vi "Abort.vi"(8 "error in (no error)":errorcluster, 11 "WAMP Client in":refnum<class "WAMP Client.lvclass">) -> (0 "error out":errorcluster, 3 "WAMP Client out":refnum<class "WAMP Client.lvclass">)   [LabVIEW 2020, in "wamplv.lvlib" / "WAMP Client.lvclass"]
uses:
  WAMP Client.lvclass
  Private/TypeDefs/WAMP Message Codes.ctl
  WAMP Client.lvclass/WAMP Client.ctl
  Private/Comm Handlers/ICommHandler/ICommHandler.lvclass
  wamplv.lvlib
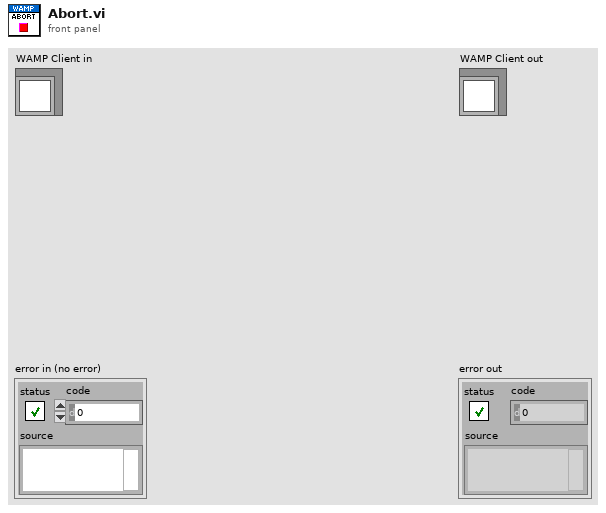
[diagram p1: front panel]
types:
  T1 = typedef "wamplv.lvlib/WAMP Message Codes.ctl" = u16
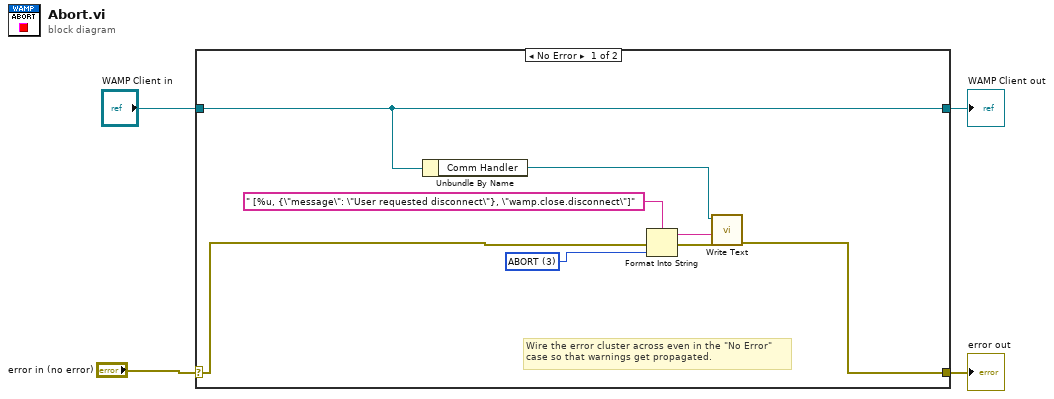
[diagram p0: block diagram]
diagram:
  n1 = case shown="No Error" "error in (no error)" {
    selector: "error in (no error)" -> [w7 w14]
    tunnel: [w5 w14] -> w3
    tunnel: [w12 w13] -> w1
    tunnel: "WAMP Client in" -> [w12 w13]
    frame No Error {
      w10 = T1 3 items=["HELLO"=1, "WELCOME"=2, "ABORT"=3, "GOODBYE"=6, "ERROR"=8, "PUBLISH"=16, "PUBLISHED"=17, "SUBSCRIBE"=32, "SUBSCRIBED"=33, "UNSUBSCRIBE"=34, "UNSUBSCRIBED"=35, "EVENT"=36, "CALL"=48, "RESULT"=59, "REGISTER"=64, "REGISTERED"=65, "UNREGISTER"=66, "UNREGISTERED"=67, "INVOCATION"=68, "YIELD"=70] ("Message Codes")
      # "Wire the error cluster across even in the \"No Error\"\ncase so that warnings get propagated."
      n2 = Unbundle By Name(w12) -> ("Comm Handler"=w9:refnum<class "ICommHandler.lvclass">)
      n3 = Format Into String(format string=" [%u, {\"message\": \"User requested disconnect\"}, \"wamp.close.disconnect\"]", error in=w7, w10) -> (resulting string=w8:string, error out=w6:errorcluster)  [unwired: 1 in]
      n4 = call-dynamic "Write Text.vi"("error in (no error)"=w6, "String"=w8, "ICommHandler in"=w9) -> ("error out"=w5:errorcluster)  [unwired: 7 in, 1 out]
    }
    frame Error {
    }
  }
  "error out" <- w3
  "WAMP Client out" <- w1
